vi "Read U32.vi"(0 "I2C In":refnum<class "I2C.lvclass">, 1 "Slave Address":u8, 5 "Register":u32, 11 "Error In":errorcluster, 12 "Register Size":T2, 13 "Byte Order":T1) -> (4 "I2C Out":refnum<class "I2C.lvclass">, 6 "Value":u32, 15 "Error Out":errorcluster)   [LabVIEW 2020, in "lv_i2c_hal.lvlib" / "I2C.lvclass"]
uses:
  I2C.lvclass
  Register Address Size.ctl
  Byte Order.ctl
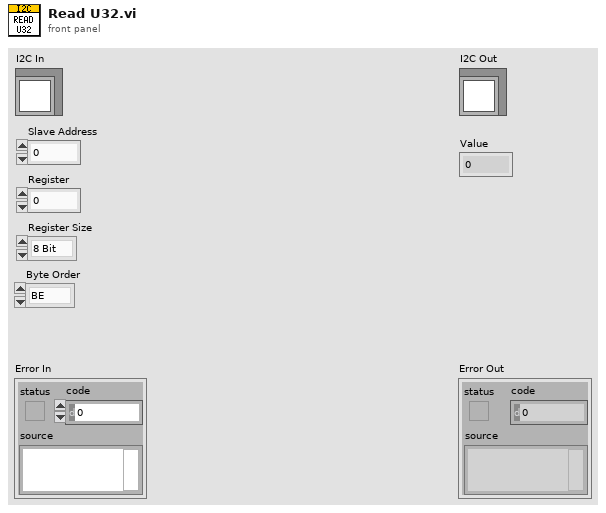
[diagram p1: front panel]
types:
  T1 = typedef "lv_i2c_hal.lvlib/I2C.lvclass/Byte Order.ctl" = enum16{"BE", "LE"}
  T2 = typedef "lv_i2c_hal.lvlib/I2C.lvclass/Register Address Size.ctl" = enum16{"8 Bit", "16 Bit", "24 Bit", "32 Bit"}
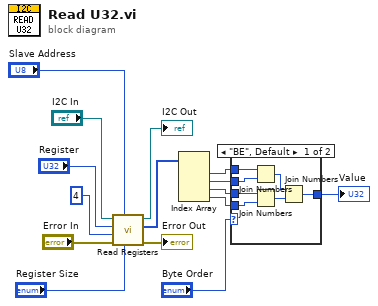
[diagram p0: block diagram]
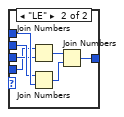
[diagram p2: hidden frame]
diagram:
  n1 = call "Read Registers.vi"("Register Size"="Register Size", "Slave Address"="Slave Address", "Error In"="Error In", "Count"=4, "Register"="Register", "I2C In"="I2C In") -> ("Error Out"=→"Error Out":errorcluster, "Values"=w12:u8[], "I2C Out"=→"I2C Out":refnum<class "I2C.lvclass">)  [unwired: 3 in]
  n2 = Index Array(array=w12) -> (element #1=w9:u8, element #2=w8:u8, element #3=w6:u8, element #4=w1:u8)  [unwired: 4 in]
  n3 = case shown="\"BE\", Default" "Byte Order" {
    tunnel: w9 -> [w19 w26]
    tunnel: w8 -> [w18 w25]
    tunnel: [w20 w29] -> w7
    tunnel: w6 -> [w17 w24]
    tunnel: w1 -> [w16 w23]
    frame "BE", Default {
      n4 = Join Numbers(hi=w19, lo=w18) -> ((hi.lo)=w22:u16)
      n5 = Join Numbers(hi=w17, lo=w16) -> ((hi.lo)=w21:u16)
      n6 = Join Numbers(hi=w22, lo=w21) -> ((hi.lo)=w20:u32)
    }
    frame "LE" {
      n7 = Join Numbers(hi=w23, lo=w24) -> ((hi.lo)=w28:u16)
      n8 = Join Numbers(hi=w25, lo=w26) -> ((hi.lo)=w27:u16)
      n9 = Join Numbers(hi=w28, lo=w27) -> ((hi.lo)=w29:u32)
    }
  }
  "Value" <- w7
